vi "Read SODA_.vi"(8 "error in (no error)":errorcluster, 11 "Nestle_Actor in":refnum<class "Nestle_Actor.lvclass">) -> (0 "error out":errorcluster, 2 "SODA?":bool, 3 "Nestle_Actor out":refnum<class "Nestle_Actor.lvclass">)   [LabVIEW 2019, in "Nestle_Actor.lvlib" / "Nestle_Actor.lvclass"]
uses:
  Nestle_Actor.lvclass
  Nestle_Actor.lvclass/Nestle_Actor.ctl
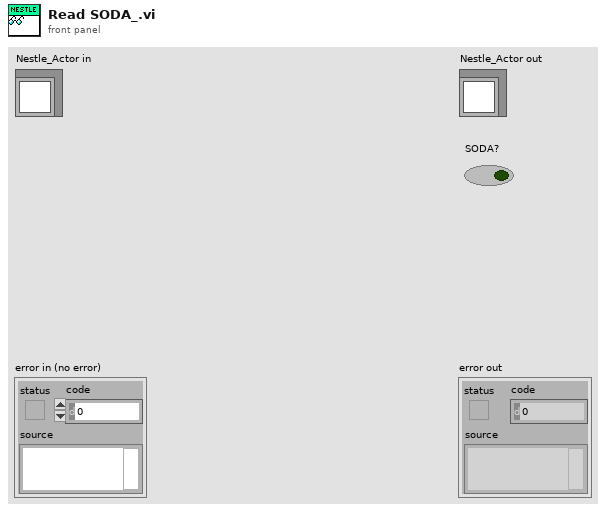
[diagram p1: front panel]
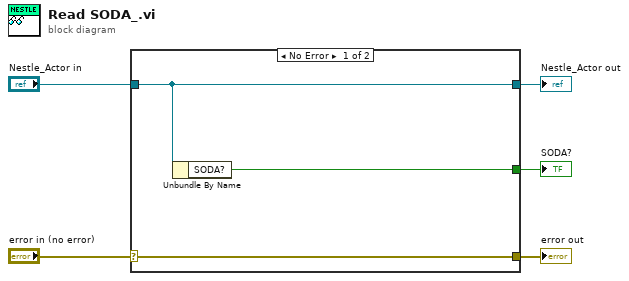
[diagram p0: block diagram]
diagram:
  n1 = case shown="No Error" "error in (no error)" {
    selector: "error in (no error)" -> [w8 w9]
    tunnel: [w8 w9] -> w4
    tunnel: [w7 w10] -> w2
    tunnel: "Nestle_Actor in" -> [w7 w10]
    tunnel: [w6 _] -> w1
    frame No Error {
      n2 = Unbundle By Name(w7) -> ("SODA?"=w6:bool)
    }
    frame Error {
    }
  }
  "error out" <- w4
  "Nestle_Actor out" <- w2
  "SODA?" <- w1
